vi "PopulateTest.vi"() -> ()   [LabVIEW 2013, in "NISE_CEF_Tests.lvlib"]
uses:
  NISE_CEF_Tests.lvlib
  Trunk/ProjectTemplates/Source/Configuration Editor Framework/Classes/cRIO/cRIO.lvclass
  Trunk/CEF_TreeControl/NISE_CEF_TreeControl.lvlib
panel:
  in  "Numeric":i32
  out "error out":errorcluster
  in  "appended path":path=path "C:/Users/bcelis.AMER/Perforce/Sales/users/BCelis/CRA/Glyphs"
  in  "View":string(tree)
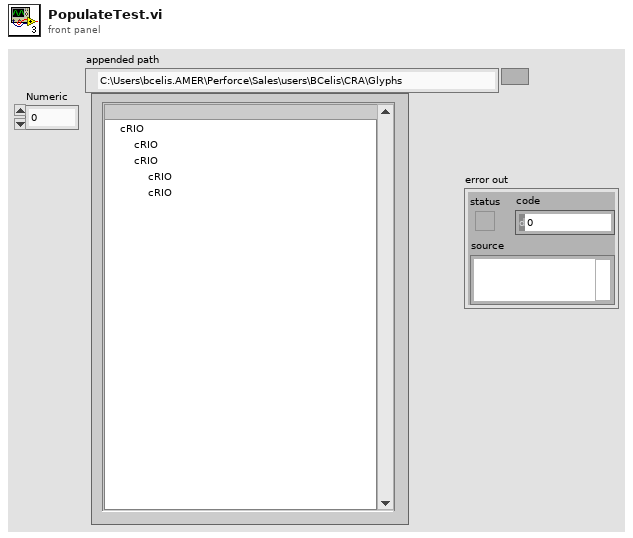
[diagram p1: front panel]
types:
  T1 = typedef "NISE_CEF_Node.lvclass/Summary.ctl" = cluster{"ID":string, "parent ID":string, "node type":string, "text":string, "additional text":string, "glyph":string, "depth":i32}
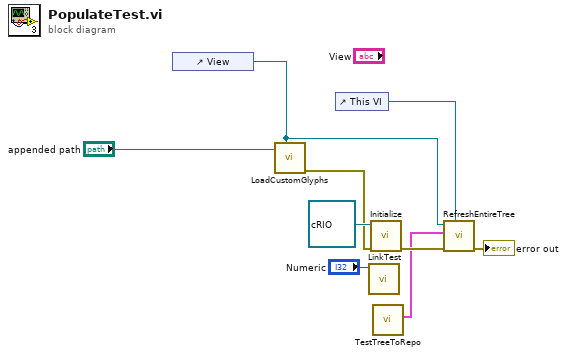
[diagram p0: block diagram]
diagram:
  n1 = control-ref of="View"() -> (w5:refnum<vi>)
  n2 = call "LoadCustomGlyphs.vi"("tree ref"=w5, "glyph directory"="appended path") -> ("error out"=w7:errorcluster)  [unwired: 9 in]
  n3 = control-ref of="This VI"() -> (w4:refnum<vi>)
  n4 = call "LinkTest.vi"("number of nodes"="Numeric") -> ()  [unwired: 10 in, 1 out]
  n5 = call-dynamic "Initialize.vi"("error in"=w7, "cRIO in"=refnum<class "cRIO.lvclass"> refnum ("cRIO.lvclass")) -> ("error out"=w6:errorcluster)  [unwired: 7 in, 2 out]
  n6 = call "TestTreeToRepo.vi"() -> ("summary"=w1:T1[])  [unwired: 11 in]
  n7 = call "RefreshEntireTree.vi"("calling VI in"=w4, "error in"=w6, "array"=w1, "tree ref in"=w5) -> ("error out"=→"error out":errorcluster)  [unwired: 7 in]
